vi "2-1.vi"(6 "停止":bool, 7 "kf(Hz/V)":dbl=50000.0, 8 "An(V)":dbl=0.02, 9 "带通Butterworth滤波器":cluster{"中心频率(Hz)":dbl, "带宽(Hz)":dbl}={"中心频率(Hz)"=150000.0, "带宽(Hz)"=220000.0}, 10 "调制信号":cluster{"fm(Hz)":dbl, "Am(V)":dbl}={"fm(Hz)"=5000.0, "Am(V)"=1.0}, 11 "载波信号":cluster{"fc(Hz)":dbl, "Ac(V)":dbl}={"fc(Hz)"=150000.0, "Ac(V)"=1.0}) -> (1 "频域":cluster{"f0":dbl, "df":dbl, "magnitude":dbl[]}(graph), 2 "时域 2":waveform(dbl)[](graph), 3 "时域":waveform(dbl)[](graph))   [LabVIEW 2018]
uses:
  <vilib>/Analysis/3filter.llb/Filter Passband Type.ctl
  <vilib>/Analysis/3filter.llb/Butterworth Filter (DBL).vi
  <vilib>/express/express analysis/Spectral/Block/exnSpectralBlock spectral measurements peak poly.vi
  <vilib>/express/express analysis/Spectral/Block/exnSpectralBlock spectral measurements peak WFM.vi
  <vilib>/express/express analysis/Spectral/XNode/ExpressSpectralMeasurementsBlockNode.xnode
  <vilib>/measure/NI_MABase.lvlib
  <vilib>/Analysis/NI_AALPro.lvlib
  <vilib>/Analysis/NI_AALBase.lvlib
panel:
  out "fh":dbl
  out "fl":dbl
  in  "选项卡控件":enum32{"调制", "滤波", "解调"}(tab)
  out "频域":cluster{"f0":dbl, "df":dbl, "magnitude":dbl[]}(graph)
  out "时域":waveform(dbl)(graph)
  out "卡森定则理论BT(Hz)":dbl
  out "数组":dbl[](array[numeric])
  out "调制信号":waveform(dbl)(graph)
  out "积分信号":waveform(dbl)(graph)
  out "采样参数（采样频率fs，采样数Ns）":cluster{dbl, dbl} {"?" format="%#_6f"; "?" format="%#_6f"}
  out "载波信号":waveform(dbl)(graph)
  # "采样率取1000*fc\n要显示n个周期的调制信号波形，\n则采样数Ns=n*fs/fm\nfh和fl为解调前滤波器\n的高和低截止频率"
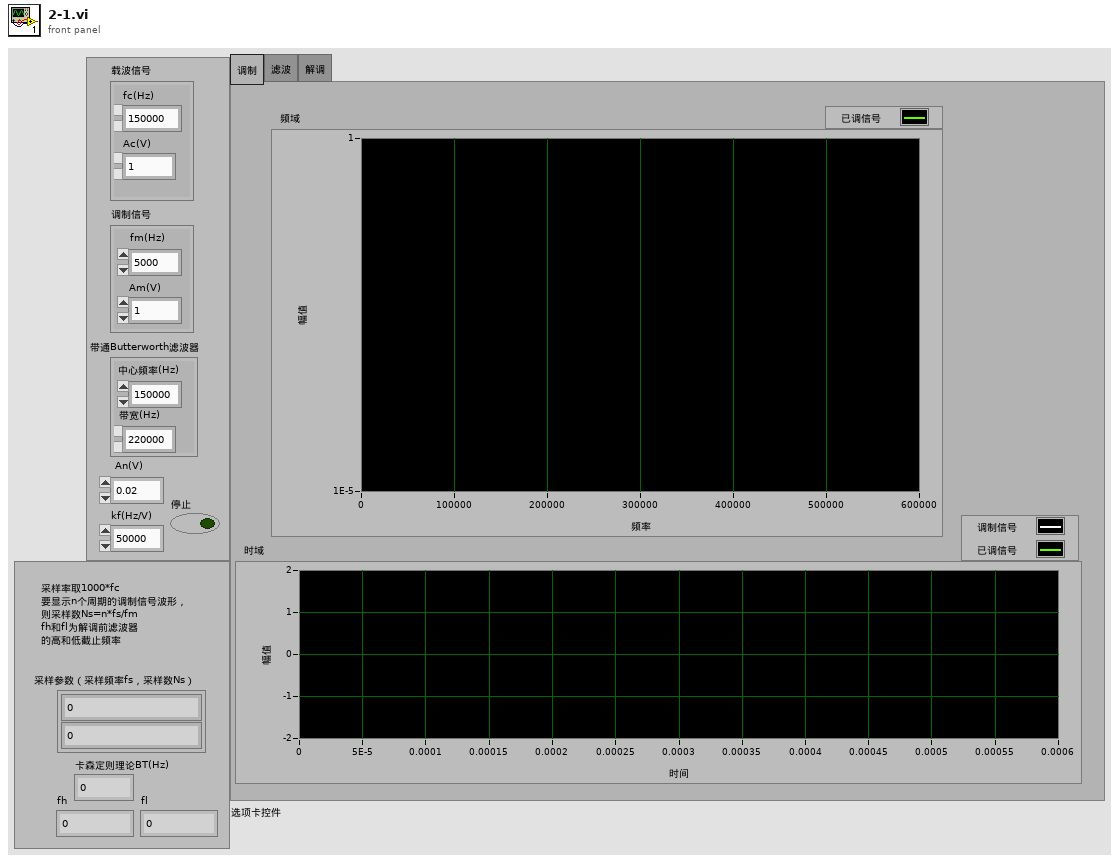
[diagram p1: front panel]
types:
  T1 = typedef "NI_AALBase.lvlib/Filter Passband Type.ctl" = enum32{"Lowpass", "Highpass", "Bandpass", "Bandstop"}
  T2 = cluster{"averaging mode":u16, "weighting mode":u16, "number of averages":u32}
  T3 = cluster{"dB On (F)":bool, "unwrap phase (F)":bool, "convert to degree (F)":bool}
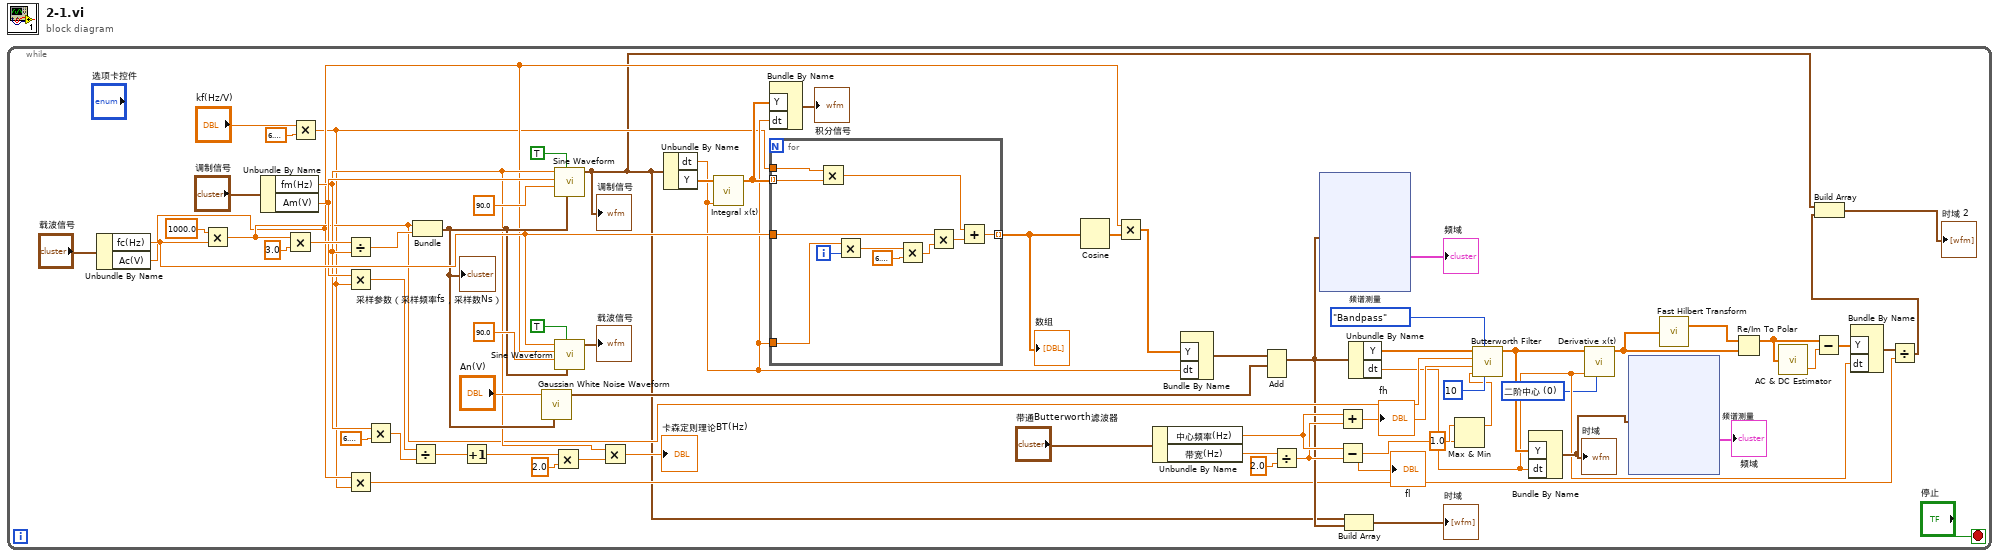
[diagram p0: block diagram]
diagram:
  n1 = while {
    stop <- "停止" stop-if-true
    w17 = u16 0 items=["二阶中心", "四阶中心", "前向", "后向"] ("method")
    n2 = Unbundle By Name("载波信号") -> ("fc(Hz)"=w55:dbl, "Ac(V)"=w13:dbl)
    n3 = Multiply(x=1000.0, y=w55) -> (x*y=w25:dbl)
    n4 = Unbundle By Name("调制信号") -> ("fm(Hz)"=w35:dbl, "Am(V)"=w42:dbl)
    n5 = Multiply(x=w25, y=3.0) -> (x*y=w63:dbl)
    n6 = Multiply(x="kf(Hz/V)", y=6.283185307179586) -> (x*y=w7:dbl)
    n7 = Divide(x=w63, y=w35) -> (x/y=w62:dbl)
    n8 = Multiply(x=w42, y=w7) -> (x*y=w40:dbl)
    n9 = Multiply(x=w13, y=w7) -> (x*y=w11:dbl)
    n10 = Multiply(x=w35, y=6.283185307179586) -> (x*y=w41:dbl)
    n11 = Divide(x=w40, y=w41) -> (x/y=w39:dbl)
    n12 = Bundle(w25, w62) -> (w49:cluster{dbl, dbl})  [unwired: 1 in]
    "采样参数（采样频率fs，采样数Ns）" <- w49
    n13 = Increment(x=w39) -> (x+1=w38:dbl)
    n14 = call <vilib>:"Gaussian White Noise Waveform.vi"("sampling info"=w49, "standard deviation"="An(V)") -> ("signal out"=w46:waveform(dbl))  [unwired: 8 in, 1 out]
    n15 = Multiply(x=w38, y=2.0) -> (x*y=w36:dbl)
    n16 = call <vilib>:"Sine Waveform.vi"("sampling info"=w49, "reset signal"=TRUE, "phase"=90.0, "amplitude"=w42, "frequency"=w35) -> ("signal out"=w5:waveform(dbl))  [unwired: 5 in, 1 out]
    "调制信号" <- w5
    n17 = call <vilib>:"Sine Waveform.vi"("sampling info"=w49, "reset signal"=TRUE, "phase"=90.0, "amplitude"=w13, "frequency"=w55) -> ("signal out"=→"载波信号":waveform(dbl))  [unwired: 5 in, 1 out]
    n18 = Multiply(x=w35, y=w36) -> (x*y=→"卡森定则理论BT(Hz)":dbl)
    n19 = Unbundle By Name(w5) -> ("dt"=w52:dbl, "Y"=w64:dbl[])
    n20 = call <vilib>:"Integral x(t).vi"("dt"=w52, "X"=w64) -> ("Integral X"=w56:dbl[])  [unwired: 8 in, 1 out]
    n21 = Bundle By Name("Y"=w56, "dt"=w52) -> (→"积分信号":waveform(dbl))  [unwired: 1 in]
    n22 = for {
      tunnel: w56 -> [w100] mode=indexing
      tunnel: w52 -> [w98]
      tunnel: w55 -> [w94]
      tunnel: [w91] -> w54 mode=indexing
      tunnel: w7 -> [w90]
      i -> [w99]
      n23 = Multiply(x=w90, y=w100) -> (x*y=w92:dbl)
      n24 = Multiply(x=w98, y=w99) -> (x*y=w96:dbl)
      n25 = Multiply(x=w96, y=6.283185307179586) -> (x*y=w95:dbl)
      n26 = Multiply(x=w94, y=w95) -> (x*y=w93:dbl)
      n27 = Add(x=w92, y=w93) -> (x+y=w91:dbl)
    }
    "数组" <- w54
    n28 = Cosine(x=w54) -> (cos(x)=w53:dbl[])
    n29 = Multiply(x=w13, y=w53) -> (x*y=w51:dbl[])
    n30 = Unbundle By Name("带通Butterworth滤波器") -> ("中心频率(Hz)"=w27:dbl, "带宽(Hz)"=w30:dbl)
    n31 = Bundle By Name("Y"=w51, "dt"=w52) -> (w48:waveform(dbl))  [unwired: 1 in]
    n32 = Add(1:w46, 2:w48) -> (0:w23:waveform(dbl))  [unwired: 1 in, 1 out]
    n33 = Divide(x=w30, y=2.0) -> (x/y=w26:dbl)
    n34 = xnode "频谱测量"("信号"=w23) -> ("FFT - （峰值）"=→"频域":cluster{"f0":dbl, "df":dbl, "magnitude":dbl[]})  [unwired: 1 in, 2 out]
    n35 = Add(x=w27, y=w26) -> (x+y=w28:dbl)
    "fh" <- w28
    n36 = Subtract(x=w27, y=w26) -> (x-y=w3:dbl)
    "fl" <- w3
    n37 = Build Array(w5, w23) -> (→"时域":waveform(dbl)[])
    n38 = Unbundle By Name(w23) -> ("Y"=w22:dbl[], "dt"=w18:dbl)
    n39 = Max & Min(x=w3, y=1.0) -> (max(x,y)=w1:dbl)  [unwired: 1 out]
    n40 = call-poly <vilib>:"Butterworth Filter.vi"("order"=10, "filter type"=Filter_Passband_Type."Bandpass", "low cutoff freq: fl"=w1, "high cutoff freq: fh"=w28, "sampling freq: fs"=w25, "X"=w22) -> ("Filtered X"=w20:dbl[])  [unwired: 2 in, 1 out]
    n41 = Bundle By Name("Y"=w20, "dt"=w18) -> (w21:waveform(dbl))  [unwired: 1 in]
    "时域" <- w21
    n42 = call <vilib>:"Derivative x(t).vi"("method"=w17, "dt"=w18, "X"=w20) -> ("dX/dt"=w10:dbl[])  [unwired: 7 in, 1 out]
    n43 = xnode "频谱测量"("信号"=w21) -> ("FFT - （峰值）"=→"频域":cluster{"f0":dbl, "df":dbl, "magnitude":dbl[]})  [unwired: 1 in, 2 out]
    n44 = call <vilib>:"Fast Hilbert Transform.vi"("X"=w10) -> ("Hilbert{X}"=w19:dbl[])  [unwired: 1 out]
    n45 = Re/Im To Polar(2:w10, 3:w19) -> (1:w16:dbl[])  [unwired: 1 out]
    n46 = call <vilib>:"AC & DC Estimator.vi"("Signal (V)"=w16) -> ("DC estimate (V)"=w15:dbl)  [unwired: 1 out]
    n47 = Subtract(x=w16, y=w15) -> (x-y=w14:dbl[])
    n48 = Bundle By Name("Y"=w14, "dt"=w18) -> (w12:waveform(dbl))  [unwired: 1 in]
    n49 = Divide(x=w12, y=w11) -> (x/y=w6:waveform(dbl))
    n50 = Build Array(w5, w6) -> (→"时域 2":waveform(dbl)[])
  }
